vi "Add.vi"(8 "error in (no error)":errorcluster, 10 "Runnable":refnum<class "Runnable.lvclass">, 11 "LUnit Test Suite In":refnum<class "LUnit Test Suite.lvclass">) -> (0 "error out":errorcluster, 3 "LUnit Test Suite Out":refnum<class "LUnit Test Suite.lvclass">)   [LabVIEW 2020, in "LUnit Test Suite.lvclass"]
doc: "Add a test method to the test suite. Order of tests will be alphabetic regardless of the order they are added to suite."
uses:
  LUnit Test Suite.lvclass
  Runnable/Runnable.lvclass
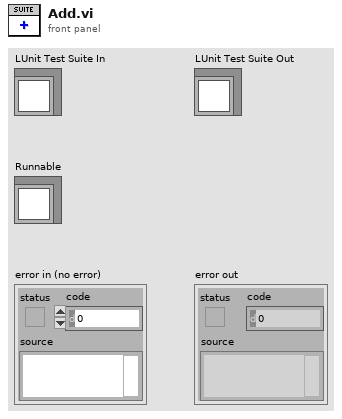
[diagram p1: front panel]
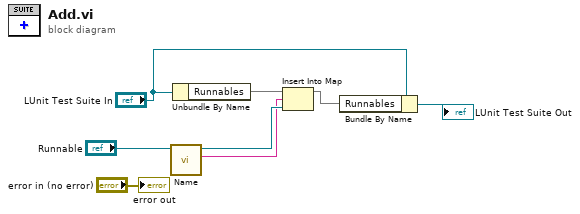
[diagram p0: block diagram]
diagram:
  n1 = call-dynamic "Name.vi"("Runnable in"="Runnable") -> ("Name"=w1:string, "Runnable out"=w2:refnum<class "Runnable.lvclass">)  [unwired: 8 in, 1 out]
  n2 = Unbundle By Name("LUnit Test Suite In") -> ("Runnables"=w5:map{string, refnum<class "Runnable.lvclass">})
  n3 = Insert Into Map(map in=w5, key=w1, value=w2) -> (map out=w4:map{string, refnum<class "Runnable.lvclass">})  [unwired: 2 out]
  n4 = Bundle By Name(cluster="LUnit Test Suite In", "Runnables"=w4) -> (→"LUnit Test Suite Out":refnum<class "LUnit Test Suite.lvclass">)
  "error out" <- "error in (no error)"
